vi "Get (Strings).vi"(5 "Tags":string[](array[string]), 7 "error in (no error)":errorcluster, 10 "ByRef Variant Repsitory in":refnum<data-value>) -> (0 "error out":errorcluster, 3 "Values":string[](array[string]))   [LabVIEW 2015, in "ByRef Variant Repository.lvlib"]
uses:
  ByRef Variant Repository.lvlib
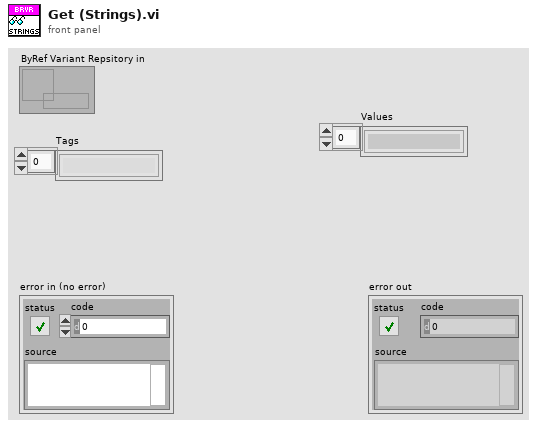
[diagram p1: front panel]
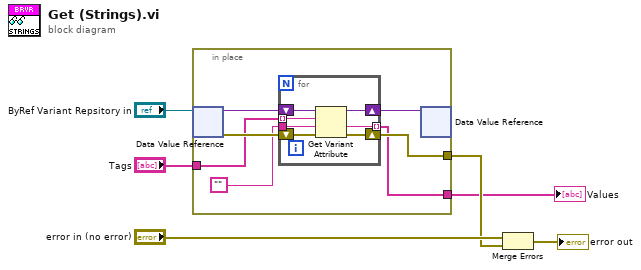
[diagram p0: block diagram]
diagram:
  n1 = in-place {
    in-place-border: [w10] -> w4
    in-place-border: "Tags" -> [w9]
    in-place-border: [w8] -> w1
    n2 = in-place-dvr #1("ByRef Variant Repsitory in") -> (w12:variant, w13:errorcluster)
    n3 = for {
      tunnel: w9 -> [w16] mode=indexing
      shift-right: [w17] -> w10
      shift-left: w13 -> [w20]
      shift-right: [w18] -> w11
      shift-left: w12 -> [w19]
      tunnel: "" ("Value") -> [w14]
      tunnel: [w15] -> w8 mode=indexing
      n4 = Get Variant Attribute(Variant=w19, name=w16, default value (empty Variant)=w14, error in=w20) -> (duplicate Variant=w18:variant, value=w15:string, error out=w17:errorcluster)  [unwired: 1 out]
    }
    n5 = in-place-dvr #1(w11) -> ()  [unwired: 2 out]
  }
  "Values" <- w1
  n6 = Merge Errors("error in (no error)", w4) -> (→"error out":errorcluster)
